vi "Run Bfr Rx - Sized Handle Rollover.vi"(4 "Data Buffer":u64, 6 "Rollover Occurred?":bool, 7 "Size Offset in":u64, 8 "error in (no error)":errorcluster, 9 "Data Size (I32)":u64, 10 "Null Offset in":u64, 11 "Data Offset in":u64) -> (0 "error out":errorcluster, 2 "Null Offset out":u64, 3 "Data Offset out":u64, 5 "Size Offset out":u64)   [LabVIEW 2019, in "UDP-Custom-Device Engine.lvlib"]
uses:
  UDP-Custom-Device Engine.lvlib
  <vilib>/NI VeriStand/VeriStand Data/Pointer Operations/Pointer.Write (I32).vi
  <vilib>/NI VeriStand/VeriStand Data/VeriStand Data.lvlib
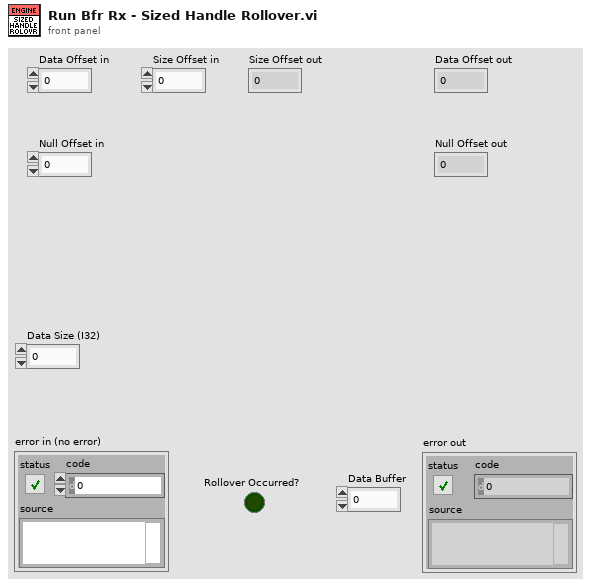
[diagram p1: front panel]
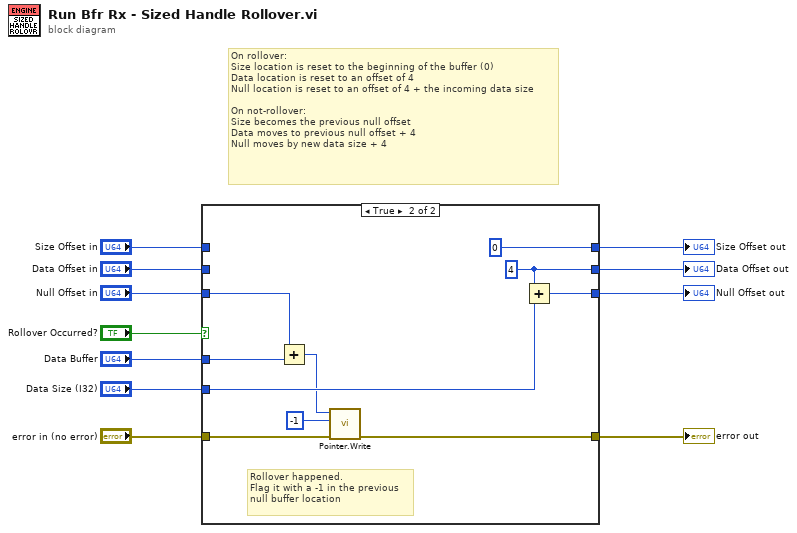
[diagram p0: block diagram]
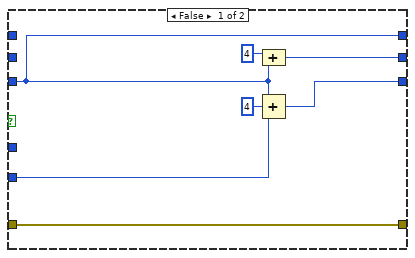
[diagram p2: hidden frame]
diagram:
  # "On rollover:\nSize location is reset to the beginning of the buffer (0)\nData location is reset to an offset of 4\nNull location is reset to an offset of 4 + the incoming data size\n\nOn not-rollover:\nSize becomes the previous null offset\nData moves to previous null offset + 4\nNull moves by new data size + 4"
  n1 = case shown="True" "Rollover Occurred?" {
    tunnel: "Data Size (I32)" -> [w14 w25]
    tunnel: "error in (no error)" -> [w18 w20]
    tunnel: "Data Buffer" -> [_ w28]
    tunnel: "Null Offset in" -> [w13 w27]
    tunnel: "Size Offset in" -> [_ _]
    tunnel: "Data Offset in" -> [_ _]
    tunnel: [w13 u64 0] -> w4
    tunnel: [w16 w24] -> w3
    tunnel: [w12 w23] -> w2
    tunnel: [w18 w19] -> w1
    frame False {
      n2 = Compound Arithmetic op=ADD(u64 4 ("value"), w13) -> (w16:u64)
      n3 = Compound Arithmetic op=ADD(w13, u64 4 ("value"), w14) -> (w12:u64)
    }
    frame True {
      w24 = u64 4
      # "Rollover happened.\nFlag it with a -1 in the previous\nnull buffer location"
      n4 = Add(x=w27, y=w28) -> (x+y=w22:u64)
      n5 = call-poly <vilib>:"Pointer.Write.vi"("error in (no error)"=w20, "value"=-1, "pointer in"=w22) -> ("error out"=w19:errorcluster)  [unwired: 6 in, 2 out]
      n6 = Add(x=w24, y=w25) -> (x+y=w23:u64)
    }
  }
  "error out" <- w1
  "Null Offset out" <- w2
  "Data Offset out" <- w3
  "Size Offset out" <- w4
